vi "Get Next Report.vi"(8 "error in":errorcluster, 9 "Last Report Number (-1)":i32=-1, 10 "Report File Pattern":string="report*", 11 "Data Directory":path) -> (0 "error out":errorcluster, 1 "New report?":bool, 2 "Report number":i32, 3 "Report Path":path)   [LabVIEW 2020, in "Waters Patrol UPLC Report Parser.lvlib" / "Instrument Manager.lvlib"]
doc: "Finds a new report, if one exists with a higher report number than the last report number given. If there are multiple new reports, it will only return the one with the highest report number. Defaults to -1, which will find any new reports."
uses:
  Instrument Manager.lvlib
  Waters Patrol UPLC Report Parser.lvlib
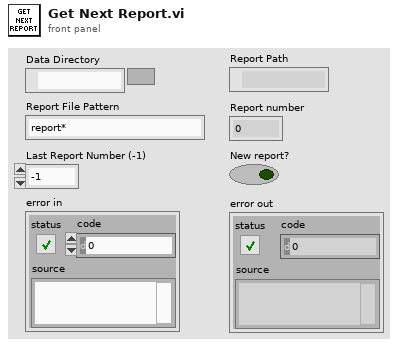
[diagram p1: front panel]
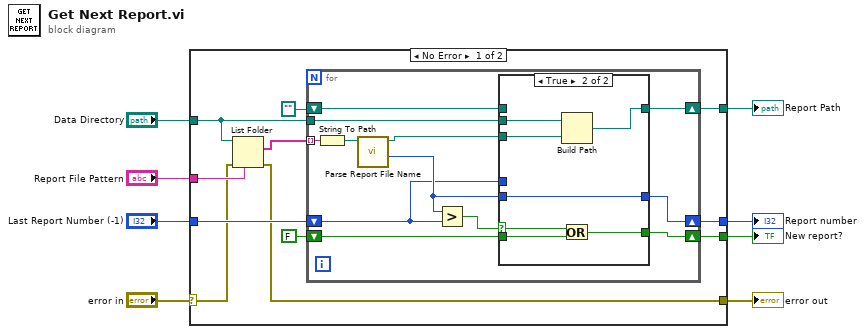
[diagram p0: block diagram]
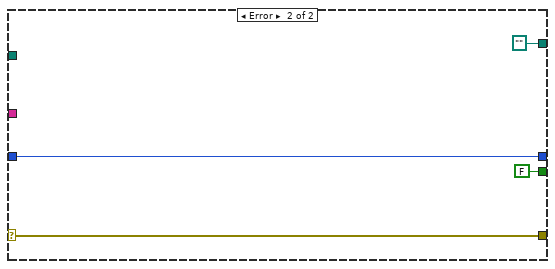
[diagram p3: hidden frame]
diagram:
  n1 = case shown="No Error" "error in" {
    selector: "error in" -> [w10 w42]
    tunnel: [w17 w44] -> w8
    tunnel: [w16 path ""] -> w7
    tunnel: [w15 FALSE] -> w6
    tunnel: "Last Report Number (-1)" -> [w14 w44]
    tunnel: "Data Directory" -> [w13 _]
    tunnel: "Report File Pattern" -> [w12 _]
    tunnel: [w9 w42] -> w1
    frame No Error {
      n2 = List Folder(path=w13, pattern=w12, error in=w10) -> (filenames=w11:string[], error out=w9:errorcluster)  [unwired: 1 in, 2 out]
      n3 = for {
        tunnel: w11 -> [w31] mode=indexing
        tunnel: w13 -> [w28]
        shift-right: [w24] -> w17
        shift-left: w14 -> [w20]
        shift-right: [w29] -> w16
        shift-left: path "" -> [w25]
        shift-right: [w22] -> w15
        shift-left: FALSE -> [w21]
        n4 = String To Path(string=w31) -> (path=w30:path)
        n5 = call "Parse Report File Name.vi"("File name"=w30) -> ("Full file name"=w27:path, "Report number"=w23:i32)  [unwired: 6 in, 2 out]
        n6 = Greater?(x=w23, y=w20) -> (0:w26:bool)
        n7 = case shown="True" w26 {
          selector: w26 -> [_ w37]
          tunnel: [w34 w41] -> w29
          tunnel: w28 -> [_ w40]
          tunnel: w27 -> [_ w39]
          tunnel: w25 -> [w34 _]
          tunnel: w20 -> [w33 _]
          tunnel: [w33 w38] -> w24
          tunnel: w23 -> [_ w38]
          tunnel: [w32 w36] -> w22
          tunnel: w21 -> [w32 w35]
          frame False {
          }
          frame True {
            n8 = Build Path(base path=w40, name or relative path=w39) -> (appended path=w41:path)
            n9 = Or(x=w37, y=w35) -> (x .or. y?=w36:bool)
          }
        }
      }
    }
    frame Error {
    }
  }
  "Report number" <- w8
  "Report Path" <- w7
  "New report?" <- w6
  "error out" <- w1
